vi "Subpanel_GetSubpanels.vi"() -> (14 "SubpanelViTable":cluster{"SectionName":string, "VIName":string}[](array[cluster]), 15 "SubpanelMainPath":path)   [LabVIEW 2016]
doc: "Init Funktion. Sucht sich die Subpanelnamen und das Verzeichnis in welchem die Panels abgelegt sind heraus. Hier erfolgt die Zuweisung zum Selection-Tree.\n\n22.08.14 / sige"
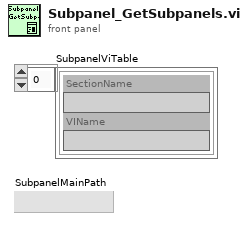
[diagram p1: front panel]
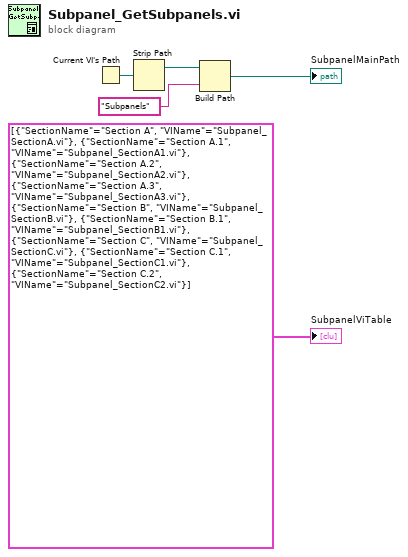
[diagram p0: block diagram]
diagram:
  n1 = Current VI's Path() -> (path=w1:path)
  n2 = Strip Path(path=w1) -> (stripped path=w2:path)  [unwired: 1 out]
  n3 = Build Path(base path=w2, name or relative path="Subpanels") -> (appended path=→"SubpanelMainPath":path)
  "SubpanelViTable" <- cluster{"SectionName":string, "VIName":string}[] [{"SectionName"="Section A", "VIName"="Subpanel_SectionA.vi"}, {"SectionName"="Section A.1", "VIName"="Subpanel_SectionA1.vi"}, {"SectionName"="Section A.2", "VIName"="Subpanel_SectionA2.vi"}, {"SectionName"="Section A.3", "VIName"="Subpanel_SectionA3.vi"}, {"SectionName"="Section B", "VIName"="Subpanel_SectionB.vi"}, {"SectionName"="Section B.1", "VIName"="Subpanel_SectionB1.vi"}, {"SectionName"="Section C", "VIName"="Subpanel_SectionC.vi"}, {"SectionName"="Section C.1", "VIName"="Subpanel_SectionC1.vi"}, {"SectionName"="Section C.2", "VIName"="Subpanel_SectionC2.vi"}]
